vi "Notify.vi"(9 "ErrorOrSuccess":refnum<class "ErrorOrSuccess.lvclass">, 10 "error in (no error)":errorcluster, 11 "Publish JSON in":refnum<class "Publish JSON.lvclass">) -> (0 "error out":errorcluster, 3 "Publish JSON out":refnum<class "Publish JSON.lvclass">)   [LabVIEW 2020, in "wamplv.lvlib" / "Publish JSON.lvclass"]
uses:
  Publish JSON.lvclass
  Message loop classes/ErrorOrSuccess/ErrorOrSuccess.lvclass
  Publish JSON.lvclass/Publish JSON.ctl
  Message loop classes/ErrorOrSuccess/ErrorOrSuccess.lvclass/ErrorOrSuccess.ctl
  Message loop classes/ErrorOrSuccess JSON/ErrorOrSuccess JSON.lvclass
  C:/local/wamplv/Private/Message loop classes/ErrorOrSuccess/ErrorOrSuccess.lvclass
  C:/local/wamplv/Private/Message loop classes/ErrorOrSuccess JSON/ErrorOrSuccess JSON.lvclass
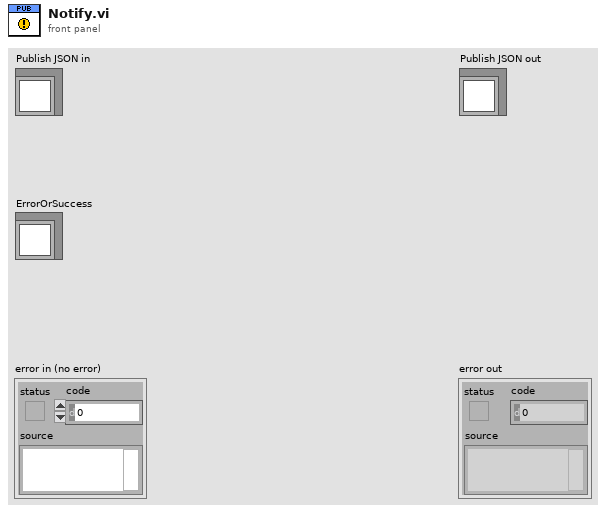
[diagram p1: front panel]
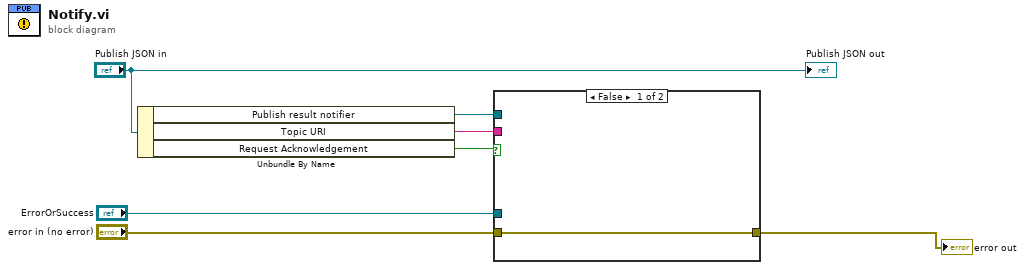
[diagram p0: block diagram]
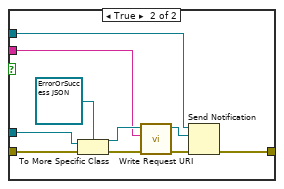
[diagram p2: hidden frame]
diagram:
  n1 = Unbundle By Name("Publish JSON in") -> ("Publish result notifier"=w2:refnum<notifier>, "Topic URI"=w4:string, "Request Acknowledgement"=w1:bool)
  n2 = case shown="False" w1 {
    tunnel: "ErrorOrSuccess" -> [_ w18]
    tunnel: "error in (no error)" -> [w8 w17]
    tunnel: w4 -> [_ w13]
    tunnel: [w8 w11] -> w3
    tunnel: w2 -> [_ w9]
    frame False {
    }
    frame True {
      n3 = To More Specific Class(target class=refnum<class "ErrorOrSuccess JSON.lvclass"> refnum ("wamplv.lvlib:ErrorOrSuccess JSON.lvclass"), reference=w18, error in=w17) -> (specific class reference=w14:refnum<class "ErrorOrSuccess JSON.lvclass">, error out=w15:errorcluster)
      n4 = call "Write Request URI.vi"("error in (no error)"=w15, "Request URI"=w13, "ErrorOrSuccess in"=w14) -> ("error out"=w12:errorcluster, "ErrorOrSuccess out"=w10:refnum<class "ErrorOrSuccess JSON.lvclass">)  [unwired: 7 in]
      n5 = Send Notification(notification=w10, notifier=w9, error in (no error)=w12) -> (error out=w11:errorcluster)  [unwired: 1 out]
    }
  }
  "error out" <- w3
  "Publish JSON out" <- "Publish JSON in"
